vi "GenerateImmediateCommand.vi"(8 "error in":errorcluster, 11 "T560Channel in":refnum<class "T560Output.lvclass">) -> (0 "error out":errorcluster, 3 "T560Channel out":refnum<class "T560Output.lvclass">)   [LabVIEW 2020, in "T560Output.lvclass"]
uses:
  T560Output.lvclass
  C:/GEECS/Developers Version/source/Device Drivers/Highland T564 DDG/SupportLibraries/DeviceSpecific/HighlandT560Lib/T560ChannelClass/T560Channel.lvclass
  T560Output.lvclass/T560Output.ctl
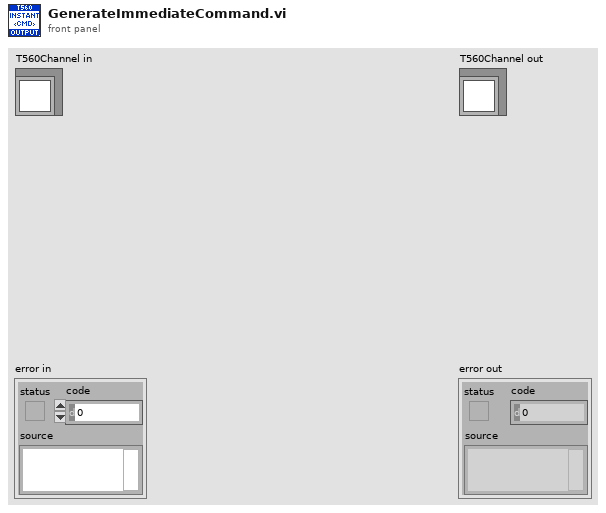
[diagram p1: front panel]
types:
  T1 = typedef "Highlandt564.lvlib/T560Channel.lvclass/ChannelName.ctl" = enum16{"Null", "A", "B", "C", "D", "Trigger"}
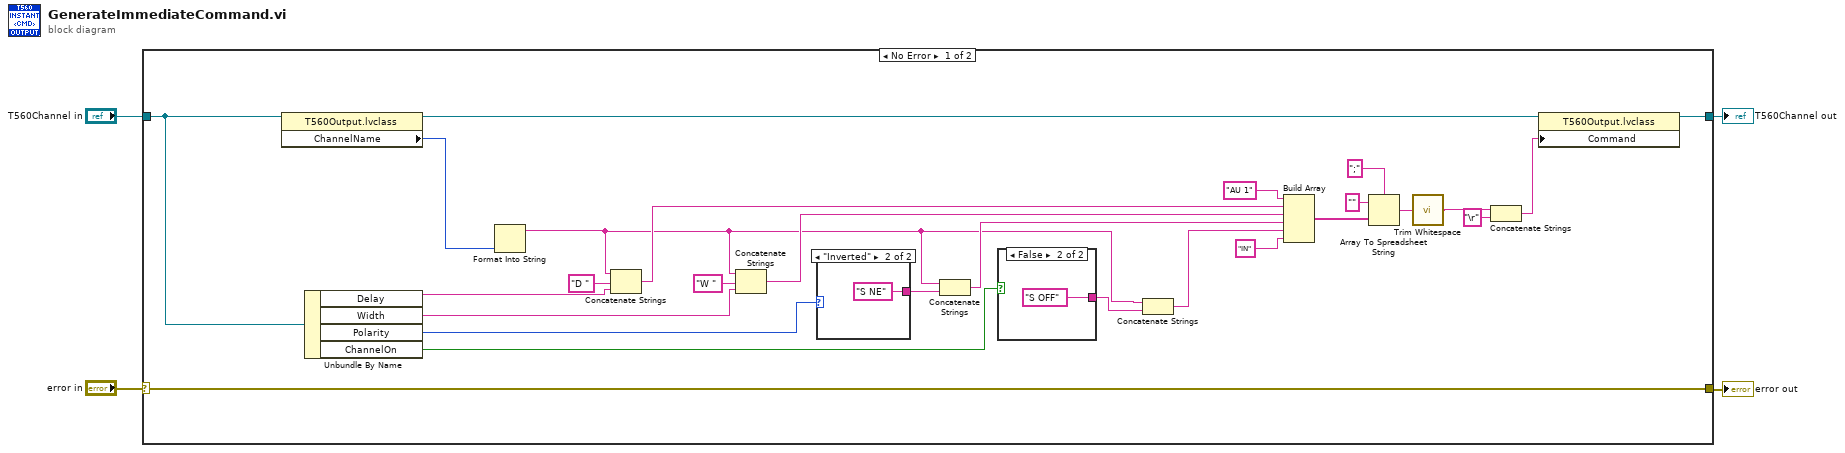
[diagram p0: block diagram]
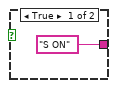
[diagram p2: hidden frame]
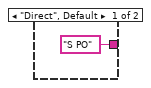
[diagram p3: hidden frame]
diagram:
  n1 = case shown="No Error" "error in" {
    selector: "error in" -> [w5 w37]
    tunnel: "T560Channel in" -> [w8 w36]
    tunnel: [w5 w37] -> w4
    tunnel: [w9 w36] -> w3
    frame No Error {
      n2 = property class="T560Output.lvclass"(reference=w8) -> (reference out=w7:refnum<class "T560Output.lvclass">, "ChannelName"=w6:T1)  [unwired: 1 in, 1 out]
      n3 = Unbundle By Name(w8) -> ("Delay"=w18:string, "Width"=w31:string, "Polarity"=w20:enum16{"Direct", "Inverted"}, "ChannelOn"=w22:bool)
      n4 = Format Into String(w6) -> (resulting string=w14:string)  [unwired: 3 in, 1 out]
      n5 = Concatenate Strings(w14, "D ", w18) -> (w26:string)
      n6 = Concatenate Strings(w14, "W ", w31) -> (w27:string)
      n7 = case shown="\"Inverted\"" w20 {
        tunnel: ["S PO" "S NE"] -> w19
        frame "Direct", Default {
        }
        frame "Inverted" {
        }
      }
      n8 = Concatenate Strings(w14, w19) -> (w21:string)
      n9 = case shown="False" w22 {
        tunnel: ["S ON" "S OFF"] -> w23
        frame True {
        }
        frame False {
        }
      }
      n10 = Concatenate Strings(w14, w23) -> (w24:string)
      n11 = Build Array("AU 1" ("element"), w26, w27, w21, w24, "IN" ("element")) -> (w28:string[])
      n12 = Array To Spreadsheet String(delimiter (Tab)=";", array=w28, 3:"" ("format string")) -> (spreadsheet string=w12:string)
      n13 = call "Trim Whitespace.vi"("string"=w12) -> ("trimmed string"=w11:string)  [unwired: 1 in]
      n14 = Concatenate Strings(w11, "\r" ("string")) -> (w10:string)
      n15 = property class="T560Output.lvclass"(reference=w7, "Command"=w10) -> (reference out=w9:refnum<class "T560Output.lvclass">)  [unwired: 1 in, 1 out]
    }
    frame Error {
    }
  }
  "error out" <- w4
  "T560Channel out" <- w3
